vi "RSZVB Set Calibration Power Meter Readings.vi"(8 "error in (no error)":errorcluster {"code" format="%.0x"}, 9 "Power Meter Readings (1)":i32=1, 11 "VISA resource name":refnum<visa-resource-name>) -> (0 "error out":errorcluster {"code" format="%.0x"}, 3 "VISA resource name out":refnum<visa-resource-name>)   [LabVIEW 2011]
doc: "This VI selects the number of power meter readings for source power calibration method \nRSZVB Set Power Calibration Method Source.vi set to RRAFter.\n\nRemote-control command(s):\nSOURce<Ch>:POWer<Pt>:CORRection:COLLect:PMReadings"
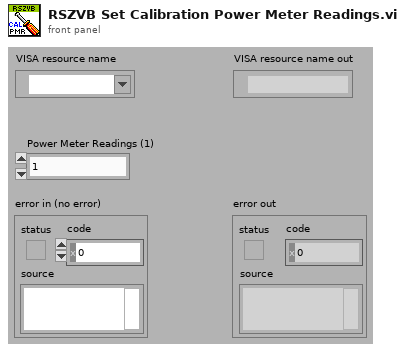
[diagram p1: front panel]
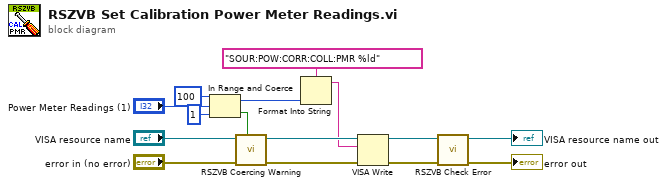
[diagram p0: block diagram]
diagram:
  n1 = In Range and Coerce(upper limit=100, x="Power Meter Readings (1)", lower limit=1) -> (coerced(x)=w1:i32, In Range?=w11:bool)
  n2 = call "RSZVB Coercing Warning.vi"("In Range?"=w11, "error in (no error)"="error in (no error)", "VISA session"="VISA resource name") -> ("error out"=w15:errorcluster, "dup VISA session"=w14:refnum<visa-resource-name>)  [unwired: 7 in]
  n3 = Format Into String(format string="SOUR:POW:CORR:COLL:PMR %ld", w1) -> (resulting string=w8:string)  [unwired: 2 in, 1 out]
  n4 = VISA Write(VISA resource name=w14, write buffer=w8, error in (no error)=w15) -> (VISA resource name out=w13:refnum<visa-resource-name>, error out=w12:errorcluster)  [unwired: 1 out]
  n5 = call "RSZVB Check Error.vi"("error in (no error)"=w12, "VISA session"=w13) -> ("error out"=→"error out":errorcluster, "dup VISA session"=→"VISA resource name out":refnum<visa-resource-name>)  [unwired: 8 in]
